vi "LV to DAT 2D.vi"(4 "append to file? (new file:F)":bool, 6 "wavenames (.Vx, etc)":string[](array[string]), 7 "filename":string, 8 "error in":errorcluster, 9 "Data":dbl[][](array[numeric]), 10 "Comments":string, 11 "path":path) -> (0 "error out":errorcluster, 3 "new file path":path)   [LabVIEW 2016, in "LV to ITX.lvclass"]
uses:
  LV to ITX.lvclass
  Typedefs/Filetype--enum.ctl
  <vilib>/Utility/file.llb/Write Delimited Spreadsheet (DBL).vi
  <vilib>/Utility/file.llb/Write Delimited Spreadsheet (string).vi
panel:
  out "appended array":string[][](array[string])
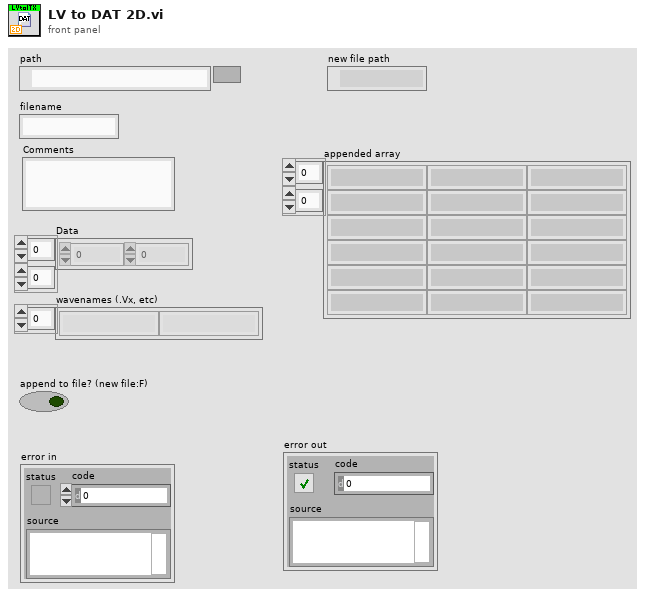
[diagram p1: front panel]
types:
  T1 = typedef "LV to ITX.lvclass/Filetype--enum.ctl" = enum16{"DAT", "ITX", "HDF5", "TDMS", "VI"}
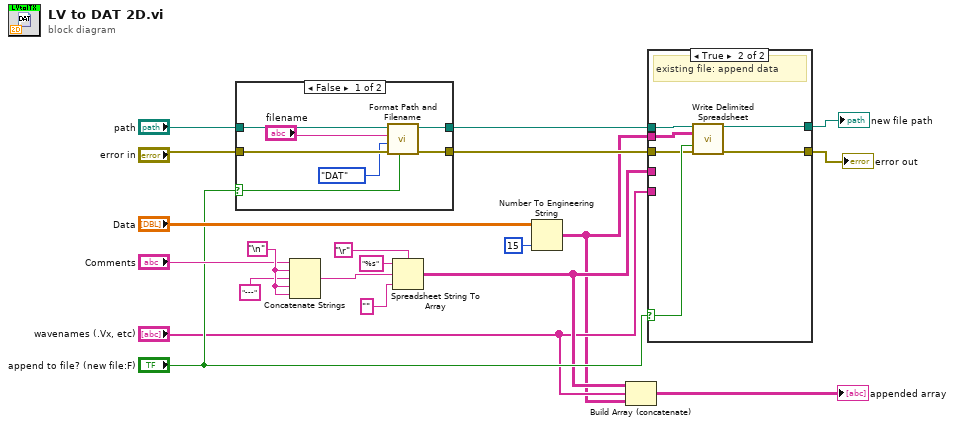
[diagram p0: block diagram]
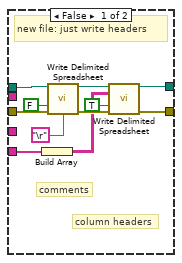
[diagram p2: hidden frame]
diagram:
  w13 = "\n"
  n1 = case shown="False" "append to file? (new file:F)" {
    selector: "append to file? (new file:F)" -> [w23 _]
    tunnel: [w21 w29] -> w9
    tunnel: "path" -> [w25 w29]
    tunnel: "error in" -> [w26 w28]
    tunnel: [w24 w28] -> w8
    frame False {
      n2 = call "Format Path and Filename.vi"("append? (F)"=w23, "error in"=w26, "Type (TDMS)"=Filetype--enum."DAT", "filename"="filename", "path"=w25) -> ("error out"=w24:errorcluster, "path"=w21:path)  [unwired: 4 in, 1 out]
    }
    frame True {
    }
  }
  n3 = Concatenate Strings("Comments", w13, "---" ("string"), w13, w13) -> (w14:string)
  n4 = Spreadsheet String To Array(delimiter (Tab)="\r", format string="%s", spreadsheet string=w14, array type (2D Dbl)="") -> (array=w4:string[][])
  n5 = Number To Engineering String(2:i16 15 ("precision (6)"), 4:"Data") -> (0:w2:string[][])  [unwired: 2 out]
  n6 = Build Array (concatenate)(w4, "wavenames (.Vx, etc)", w2) -> (→"appended array":string[][])
  n7 = case shown="True" "append to file? (new file:F)" {
    selector: "append to file? (new file:F)" -> [_ w45]
    tunnel: [w38 w43] -> w6
    tunnel: w9 -> [w40 w46]
    tunnel: w8 -> [w39 w44]
    tunnel: [w35 w42] -> w7
    tunnel: w2 -> [_ w41]
    tunnel: "wavenames (.Vx, etc)" -> [w30 _]
    tunnel: w4 -> [_ _]
    frame False {
      # "column headers"
      # "comments"
      # "new file: just write headers"
      n8 = Build Array(w30) -> (w31:string[][])
      n9 = call-poly <vilib>:"Write Delimited Spreadsheet.vi"("file path (dialog if empty)"=w40, "append to file? (new file:F)"=FALSE, "error in (no error)"=w39, "delimiter (\\t)"="\r") -> ("new file path (Not A Path if cancelled)"=w36:path, "error out"=w37:errorcluster)  [unwired: 10 in]
      n10 = call-poly <vilib>:"Write Delimited Spreadsheet.vi"("file path (dialog if empty)"=w36, "2D data"=w31, "append to file? (new file:F)"=TRUE, "error in (no error)"=w37) -> ("new file path (Not A Path if cancelled)"=w38:path, "error out"=w35:errorcluster)  [unwired: 10 in]
    }
    frame True {
      # "existing file: append data"
      n11 = call-poly <vilib>:"Write Delimited Spreadsheet.vi"("file path (dialog if empty)"=w46, "2D data"=w41, "append to file? (new file:F)"=w45, "error in (no error)"=w44) -> ("new file path (Not A Path if cancelled)"=w43:path, "error out"=w42:errorcluster)  [unwired: 10 in]
    }
  }
  "new file path" <- w6
  "error out" <- w7
